vi "mix time and date array.vi"(11 "Array in":string[][](array[string])) -> (3 "Array out":timestamp[](array[timestamp]))   [LabVIEW 2018]
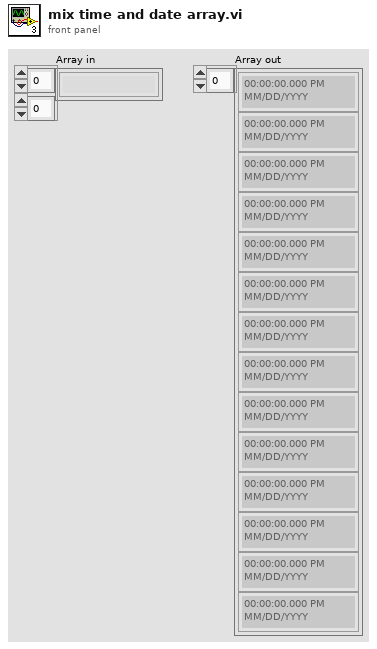
[diagram p1: front panel]
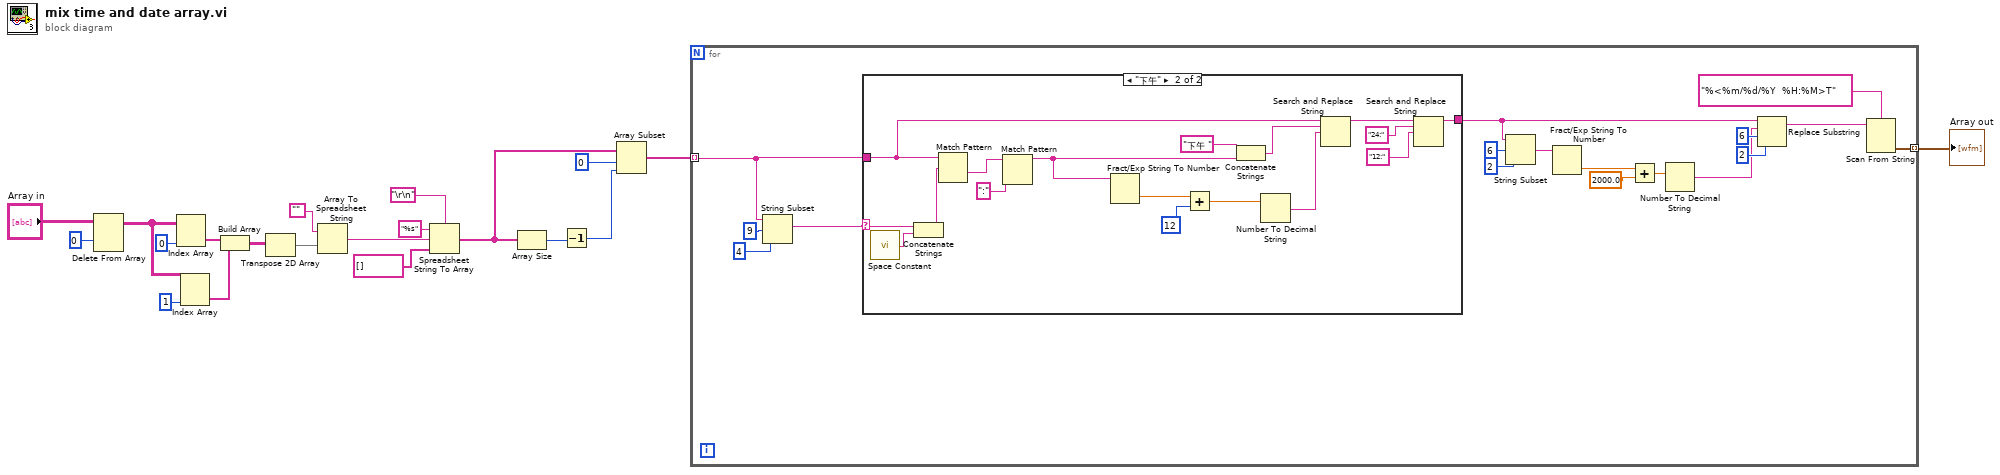
[diagram p0: block diagram]
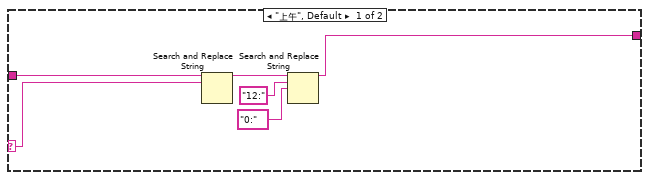
[diagram p2: hidden frame]
diagram:
  n1 = Delete From Array(array="Array in", index (row)=0) -> (array with subset deleted=w2:string[][])  [unwired: 2 in, 1 out]
  n2 = Index Array(array=w2, index (col)=0 ("disabled index (col)")) -> (element=w3:string[])  [unwired: 1 in]
  n3 = Index Array(array=w2, index (col)=1 ("disabled index (col)")) -> (element=w4:string[])  [unwired: 1 in]
  n4 = Build Array(w3, w4) -> (w5:string[][])
  n5 = Transpose 2D Array(2D array=w5) -> (transposed array=w6:string[][])
  n6 = Array To Spreadsheet String(array=w6, 3:"") -> (spreadsheet string=w7:string)  [unwired: 1 in]
  n7 = Spreadsheet String To Array(delimiter (Tab)="\r\n", format string="%s", spreadsheet string=w7, array type (2D Dbl)=string[] []) -> (array=w8:string[])
  n8 = Array Size(array=w8) -> (size(s)=w9:i32)
  n9 = Decrement(x=w9) -> (x-1=w10:i32)
  n10 = Array Subset(array=w8, index=0, length=w10) -> (w11:string[])
  n11 = for {
    tunnel: w11 -> [w34] mode=indexing
    tunnel: [w22] -> w1 mode=indexing
    n12 = String Subset(string=w34, offset (0)=9, length (rest)=4 ("length (rest)")) -> (substring=w35:string)
    n13 = case shown="\"下午\"" w35 {
      selector: w35 -> [w43 w60]
      tunnel: [w39 w45] -> w31
      tunnel: w34 -> [w38 w50]
      frame "上午", Default {
        n14 = Search and Replace String(input string=w38, search string=w43) -> (result string=w42:string)  [unwired: 6 in, 3 out]
        n15 = Search and Replace String(input string=w42, search string="12:", replace string="0:") -> (result string=w39:string)  [unwired: 5 in, 3 out]
      }
      frame "下午" {
        n16 = call <vilib>:"Space Constant.vi"() -> ("String"=w59:string)
        n17 = Concatenate Strings(w60, w59) -> (w58:string)
        n18 = Match Pattern(string=w50, regular expression=w58) -> (after substring=w57:string)  [unwired: 1 in, 3 out]
        n19 = Match Pattern(string=w57, regular expression=":") -> (before substring=w44:string)  [unwired: 1 in, 3 out]
        n20 = Fract/Exp String To Number(string=w44) -> (number=w49:dbl)  [unwired: 3 in, 1 out]
        n21 = Add(x=w49, y=12) -> (x+y=w54:dbl)
        n22 = Concatenate Strings("下午 ", w44) -> (w52:string)
        n23 = Number To Decimal String(number=w54) -> (decimal integer string=w51:string)  [unwired: 1 in]
        n24 = Search and Replace String(input string=w50, search string=w52, replace string=w51) -> (result string=w48:string)  [unwired: 5 in, 3 out]
        n25 = Search and Replace String(input string=w48, search string="24:", replace string="12:") -> (result string=w45:string)  [unwired: 5 in, 3 out]
      }
    }
    n26 = String Subset(string=w31, offset (0)=6, length (rest)=2 ("length (rest)")) -> (substring=w28:string)
    n27 = Fract/Exp String To Number(string=w28) -> (number=w27:dbl)  [unwired: 3 in, 1 out]
    n28 = Add(x=w27, y=2000.0) -> (x+y=w25:dbl)
    n29 = Number To Decimal String(number=w25) -> (decimal integer string=w24:string)  [unwired: 1 in]
    n30 = Replace Substring(2:2 ("length (len. of substring)"), 3:6 ("offset (0)"), 4:w24, 5:w31) -> (1:w23:string)  [unwired: 1 out]
    n31 = Scan From String(format string="%<%m/%d/%Y  %H:%M>T", input string=w23) -> (output 1=w22:timestamp)  [unwired: 3 in, 3 out]
  }
  "Array out" <- w1
